vi "Selected Index Read.vi"(4 "error in (no error)":errorcluster, 6 "Container State":T2, 7 "Display State In":T1) -> (0 "error out":errorcluster, 2 "Value":i32[](array[numeric]), 3 "Display State Out":T1)   [LabVIEW 2014, in "ListBox XControl.xctl"]
uses:
  ListBox XControl.xctl
  <vilib>/_xctls/Container State.ctl
  State ListBox.ctl
  <vilib>/_xctls/XControlSupport.lvlib
panel:
  # "Replace the Value Indicator below with an Indicator of desired type.\nDo not remove this Indicator or the others from the connector pane. \nDo not change the connector pane pattern.\nThe Value Indicator should always be the second terminal from top on the output side in the connector pane."
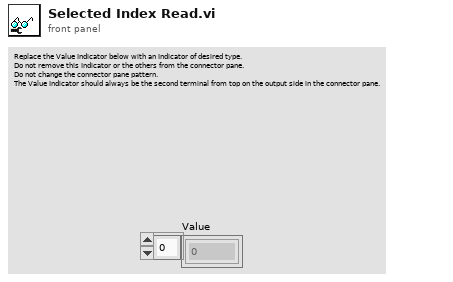
[diagram p1: front panel]
types:
  T1 = typedef "ListBox XControl.xctl/State ListBox.ctl" = cluster{"ItemNames[]":string[], "Listbox Ref":refnum<vi>, "Select All By Default":bool}
  T2 = typedef "XControlSupport.lvlib/Container State.ctl" = cluster{"Indicator?":bool, "Run Mode?":bool, " Refnum":refnum<vi>}
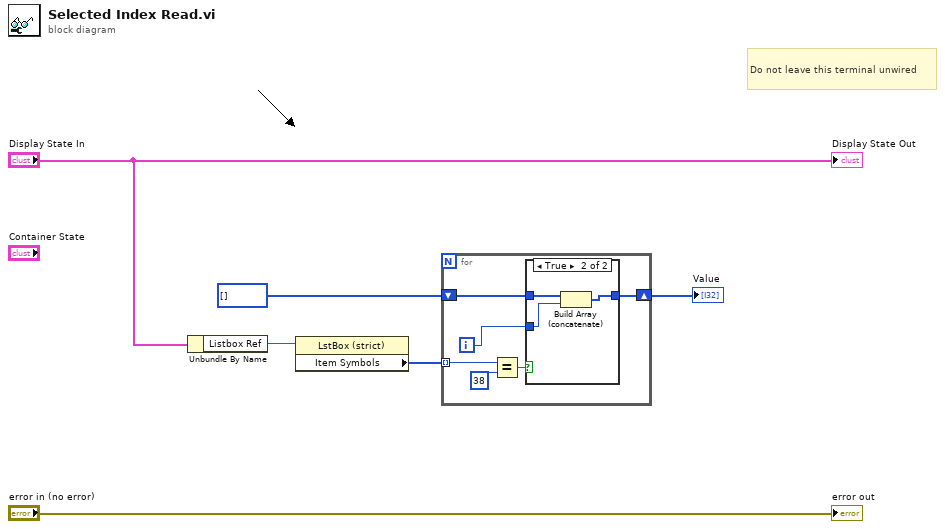
[diagram p0: block diagram]
diagram:
  # "Do not leave this terminal unwired"
  n1 = Unbundle By Name("Display State In") -> ("Listbox Ref"=w5:refnum<vi>)
  n2 = property class="LstBox (strict)"(reference=w5) -> ("Item Symbols"=w4:i32[])  [unwired: 1 in, 2 out]
  n3 = for {
    shift-right: [w8] -> w1
    shift-left: i32[] [] ("ItemNames[]") -> [w9]
    tunnel: w4 -> [w12] mode=indexing
    i -> [w7]
    n4 = Equal?(x=w12, y=38) -> (x = y?=w10:bool)
    n5 = case shown="True" w10 {
      tunnel: w9 -> [w13 w15]
      tunnel: w7 -> [_ w16]
      tunnel: [w13 w14] -> w8
      frame False {
      }
      frame True {
        n6 = Build Array (concatenate)(w15, w16) -> (w14:i32[])
      }
    }
  }
  "Value" <- w1
  "error out" <- "error in (no error)"
  "Display State Out" <- "Display State In"
